vi "CheckTwoArrayEqual.vi"(1 "´¡¥óÂI«H®§":string[][](array[string]), 2 "´¡¥óÂI«H®§(¤w¦sÀÉ)":string[][](array[string])) -> (0 "Equal¡H":bool)   [LabVIEW 2014]
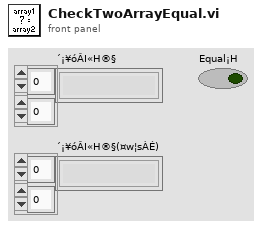
[diagram p1: front panel]
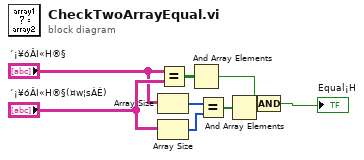
[diagram p0: block diagram]
diagram:
  n1 = Array Size(array="´¡¥óÂI«H®§") -> (size(s)=w2:i32[])
  n2 = Array Size(array="´¡¥óÂI«H®§(¤w¦sÀÉ)") -> (size(s)=w3:i32[])
  n3 = Equal?(x="´¡¥óÂI«H®§", y="´¡¥óÂI«H®§(¤w¦sÀÉ)") -> (x = y?=w1:bool[][])
  n4 = And Array Elements(Boolean array=w1) -> (logical AND=w5:bool)
  n5 = Equal?(x=w2, y=w3) -> (x = y?=w4:bool[])
  n6 = And Array Elements(Boolean array=w4) -> (logical AND=w6:bool)
  n7 = Compound Arithmetic op=AND(w5, w6) -> (→"Equal¡H":bool)
